vi "Scanner_Mirror_configuration.vi"(0 "POS X":dbl, 1 "POS Y":dbl, 2 "POS Z":dbl, 5 "error in":errorcluster) -> (19 "error out":errorcluster)   [LabVIEW 2011]
uses:
  Utilities/controls/ctlSeqFNs_PI_SysNr.ctl
  Variables/GlobalSetConfigurationPhysikalInstruments.vi
  Variables/GlobalSetNumberOfDigits_Scanners.vi
  Variables/GlobalSetGetPositionParameters.vi
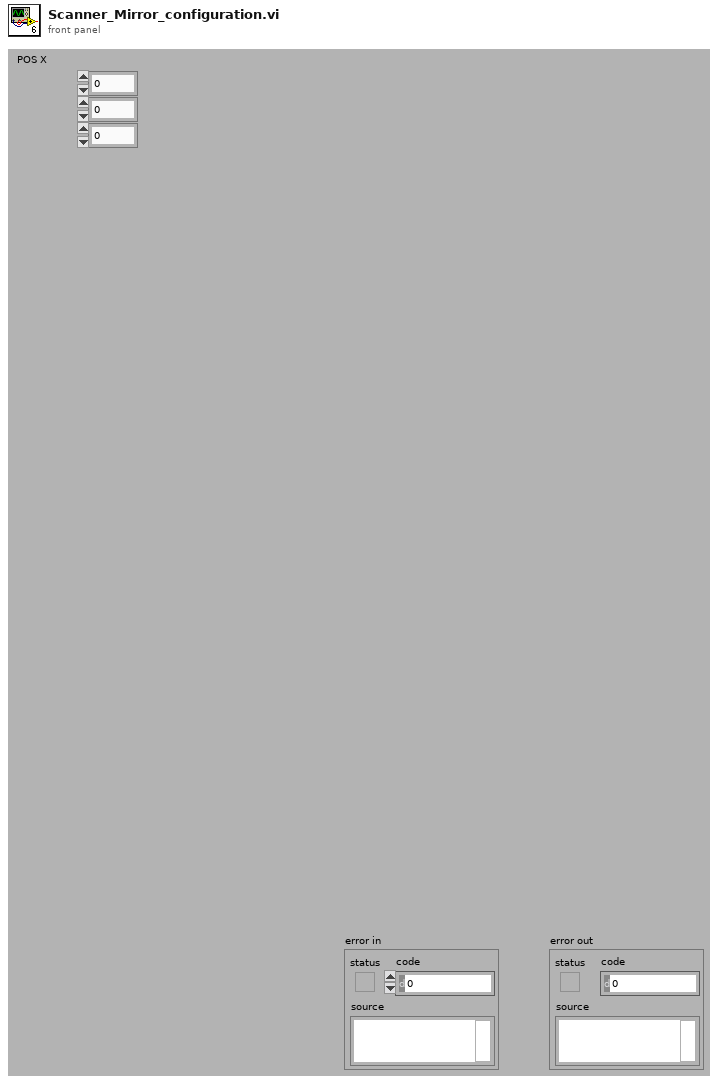
[diagram p1: front panel]
types:
  T1 = typedef "ctlSeqFNs_PI_SysNr.ctl" = enum16{"Zero", "E517", "E710"}
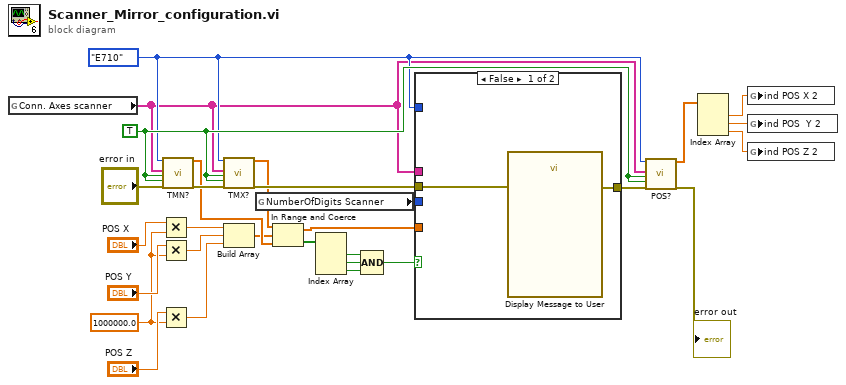
[diagram p0: block diagram]
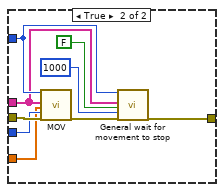
[diagram p2: hidden frame]
diagram:
  w17 = 1000000.0 ("y")
  w15 = ctlSeqFNs_PI_SysNr."E710" ("DeviceNr.")
  w28 = TRUE ("All axes?")
  n1 = global read "GlobalSetConfigurationPhysikalInstruments.vi" "Conn. Axes scanner"() -> (w14:string[])
  n2 = Multiply(x="POS X", y=w17) -> (x*y=w25:dbl)
  n3 = Multiply(x="POS Y", y=w17) -> (x*y=w24:dbl)
  n4 = Multiply(x="POS Z", y=w17) -> (x*y=w23:dbl)
  n5 = call "TMN?.vi"("System no."=w15, "Axes to query"=w14, "All axes?"=w28, "Axis identifier?"=w28, "error in"="error in") -> ("Minimum travel limit"=w9:dbl[], "error out"=w27:errorcluster)  [unwired: 13 in]
  n6 = call "TMX?.vi"("System no."=w15, "Axes to query"=w14, "All axes?"=w28, "Axis identifier?"=w28, "error in"=w27) -> ("Maximum travel limit"=w8:dbl[], "error out"=w29:errorcluster)  [unwired: 13 in]
  n7 = Build Array(w25, w24, w23) -> (w7:dbl[])
  n8 = global read "GlobalSetNumberOfDigits_Scanners.vi" "NumberOfDigits Scanner"() -> (w19:i32)
  n9 = In Range and Coerce(upper limit=w8, x=w7, lower limit=w9) -> (coerced(x)=w6:dbl[], In Range?=w13:bool[])
  n10 = Index Array(array=w13) -> (element #1=w12:bool, element #2=w11:bool, element #3=w10:bool)  [unwired: 3 in]
  n11 = Compound Arithmetic op=AND(w12, w11, w10) -> (w5:bool)
  n12 = case shown="False" w5 {
    tunnel: w29 -> [w30 w40]
    tunnel: w19 -> [_ w39]
    tunnel: [w31 w35] -> w16
    tunnel: w15 -> [_ w34]
    tunnel: w14 -> [_ w33]
    tunnel: w6 -> [_ w32]
    frame False {
      n13 = call "Display Message to User"("error in (no error)"=w30) -> ("error out"=w31:errorcluster)  [unwired: 9 in, 1 out]
    }
    frame True {
      n14 = call "MOV.vi"("System no."=w34, "Axes to move"=w33, "Position values"=w32, "No.of digits"=w39, "error in"=w40) -> ("error out"=w36:errorcluster)  [unwired: 14 in]
      n15 = call "General wait for movement to stop.vi"("System no."=w34, "Axes to wait for"=w33, "All axes?"=FALSE, "Additional wait time, ms"=u32 1000, "error in"=w36) -> ("error out"=w35:errorcluster)  [unwired: 13 in, 1 out]
    }
  }
  n16 = call "POS?.vi"("System no."=w15, "Axes to query"=w14, "All axes?"=w28, "Axis identifier?"=w28, "error in"=w16) -> ("Position"=w4:dbl[], "error out"=→"error out":errorcluster)  [unwired: 13 in]
  n17 = Index Array(array=w4) -> (element #1=w3:dbl, element #2=w2:dbl, element #3=w1:dbl)  [unwired: 3 in]
  n18 = global write "GlobalSetGetPositionParameters.vi" "ind POS X 2"(w3) -> ()
  n19 = global write "GlobalSetGetPositionParameters.vi" "ind POS  Y 2"(w2) -> ()
  n20 = global write "GlobalSetGetPositionParameters.vi" "ind POS Z 2"(w1) -> ()
